vi "Encode.vi"(8 "Error In":errorcluster, 10 "Data":string, 11 "reference in":refnum<class "EncryptionDecorator.lvclass">) -> (0 "Error Out":errorcluster, 2 "Return(STRING)":string, 3 "reference in":refnum<class "EncryptionDecorator.lvclass">)   [LabVIEW 2020, in "EncryptionDecorator.lvclass"]
uses:
  EncryptionDecorator.lvclass
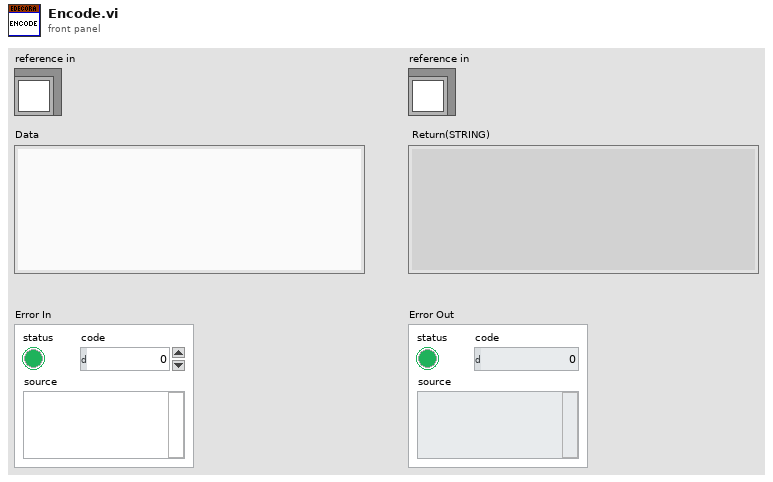
[diagram p1: front panel]
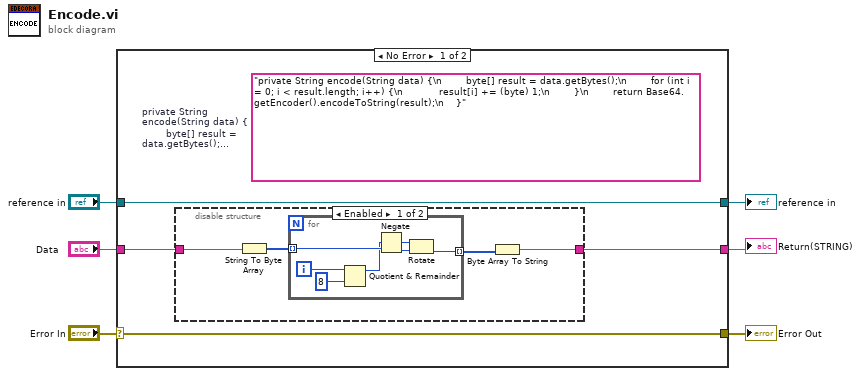
[diagram p0: block diagram]
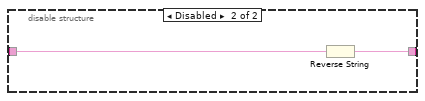
[diagram p2: hidden frame]
diagram:
  n1 = case shown="No Error" "Error In" {
    selector: "Error In" -> [w8 w24]
    tunnel: [w8 w24] -> w5
    tunnel: [w10 w23] -> w3
    tunnel: "reference in" -> [w10 w23]
    tunnel: "Data" -> [w9 _]
    tunnel: [w7 _] -> w1
    frame No Error {
      (unwired) "private String encode(String data) {\n        byte[] result = data.getBytes();\n        for (int i = 0; i < result.length; i++) {\n            result[i] += (byte) 1;\n        }\n        return Base64.getEncoder().encodeToString(result);\n    }"  # private String encode(String data) {         byte[] result = data.getBytes();         for (int i = 0; i < result.length; i++) {             result[i] += (byte) 1;         }         return Base64.getEncoder().encodeToString(result);     }
      n2 = disable-structure shown="Enabled" {
        disable-tunnel: w9 -> [w14 w21]
        disable-tunnel: [w13 w22] -> w7
        frame Enabled {
          n3 = String To Byte Array(string=w14) -> (unsigned byte array=w11:u8[])
          n4 = for {
            tunnel: w11 -> [w18] mode=indexing
            tunnel: [w17] -> w12 mode=indexing
            i -> [w20]
            n5 = Quotient & Remainder(x=w20, y=8) -> (x-y*floor(x/y)=w16:i32)  [unwired: 1 out]
            n6 = Negate(x=w16) -> (-x=w15:i32)
            n7 = Rotate(1:w18, 2:w15) -> (0:w17:u8)
          }
          n8 = Byte Array To String(unsigned byte array=w12) -> (string=w13:string)
        }
        frame Disabled {
          n9 = Reverse String(1:w21) -> (0:w22:string)
        }
      }
    }
    frame Error {
    }
  }
  "Error Out" <- w5
  "reference in" <- w3
  "Return(STRING)" <- w1
